vi "测试-Z值判定.vi"() -> ()   [LabVIEW 2018]
uses:
  <vilib>/Utility/NIReport.llb/Report Type.ctl
  <vilib>/Utility/NIReport.llb/Append Report Text (str wrap).vi
  <vilib>/addons/_office/word.llb/Word Edit Cell (str).vi
  <vilib>/Utility/NIReport.llb/NI_report.lvclass
  <vilib>/Utility/NIReport.llb/NI_ReportGenerationCore.lvlib
  <vilib>/Utility/NIReport.llb/Word/NI_Word.lvclass
  <vilib>/addons/_office/NI_ReportGenerationToolkit.lvlib
panel:
  out "报告生成路径":path
  in  "产品序号":string
  out "字符串":string
  in  "Z值":dbl[](array[numeric])
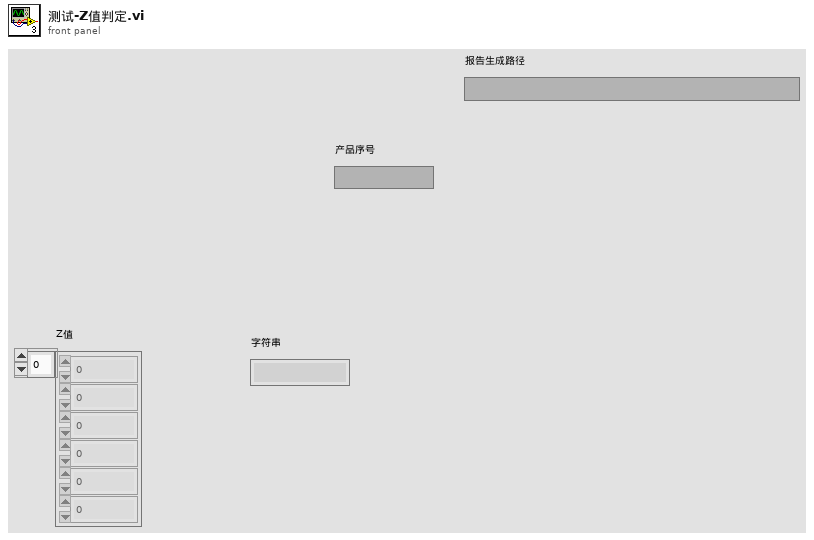
[diagram p1: front panel]
types:
  T1 = cluster{"position (Excel)":cluster{"row":i32, "column":i32}, "name (Excel)":string, "bookmark (Word)":string}
  T2 = typedef "NI_ReportGenerationCore.lvlib/Report Type.ctl" = enum16{"HTML", "Word", "Excel"}
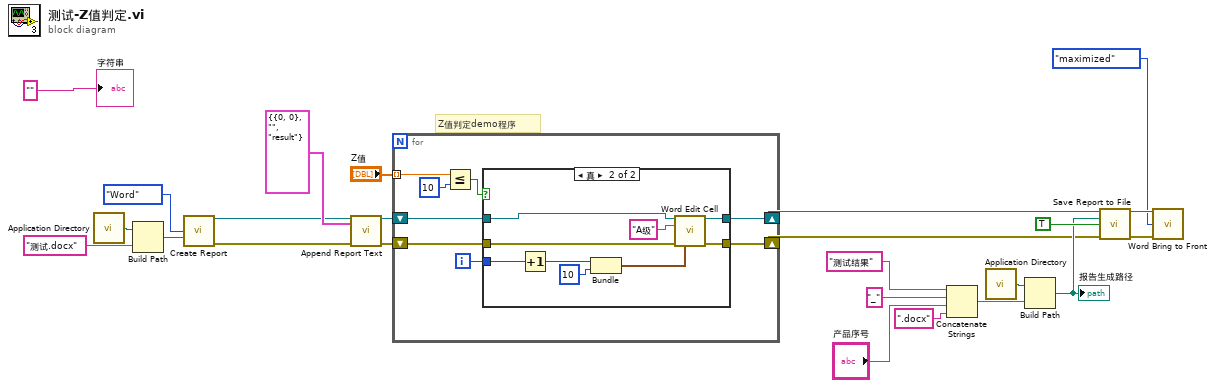
[diagram p0: block diagram]
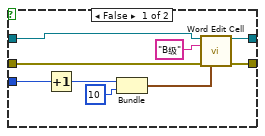
[diagram p2: hidden frame]
diagram:
  # "Z值判定demo程序"
  n1 = call <vilib>:"Application Directory.vi"() -> ("Application Directory"=w21:path)
  n2 = Build Path(base path=w21, name or relative path="测试.docx") -> (appended path=w24:path)
  n3 = call <vilib>:"Create Report.vi"("report type"=Report_Type."Word" ("Report Type"), "template (empty)"=w24) -> ("report out"=w6:refnum<class "NI_report.lvclass">, "error out"=w5:errorcluster)  [unwired: 12 in]
  n4 = call-poly <vilib>:"Append Report Text.vi"("report in"=w6, "MS Office parameters"=T1 {"position (Excel)"={"row"=0, "column"=0}, "name (Excel)"="", "bookmark (Word)"="result"}, "error in (no error)"=w5) -> ("report out"=w3:refnum<class "NI_report.lvclass">, "error out"=w4:errorcluster)  [unwired: 9 in, 2 out]
  n5 = for {
    shift-right: [w25] -> w2
    shift-left: w3 -> [w28]
    shift-right: [w26] -> w1
    shift-left: w4 -> [w27]
    tunnel: "Z值" -> [w31] mode=indexing
    i -> [w29]
    n6 = Less Or Equal?(x=w31, y=10) -> (x <= y?=w30:bool)
    n7 = case shown="真" w30 {
      tunnel: w29 -> [w35 w48]
      tunnel: w28 -> [w36 w47]
      tunnel: w27 -> [w37 w46]
      tunnel: [w34 w45] -> w26
      tunnel: [w33 w44] -> w25
      frame False {
        n8 = Increment(x=w35) -> (x+1=w41:i32)
        n9 = Bundle(w41, "y"=10) -> (w38:cluster{i32, "y":i32})  [unwired: 1 in]
        n10 = call-poly <vilib>:"Word Edit Cell.vi"("report in"=w36, "value"="B级", "error in (no error)"=w37, "start (0, 0)"=w38) -> ("report out"=w33:refnum<class "NI_report.lvclass">, "error out"=w34:errorcluster)  [unwired: 10 in]
      }
      frame True {
        n11 = Increment(x=w48) -> (x+1=w50:i32)
        n12 = Bundle(w50, "y"=10) -> (w42:cluster{i32, "y":i32})  [unwired: 1 in]
        n13 = call-poly <vilib>:"Word Edit Cell.vi"("report in"=w47, "value"="A级", "error in (no error)"=w46, "start (0, 0)"=w42) -> ("report out"=w44:refnum<class "NI_report.lvclass">, "error out"=w45:errorcluster)  [unwired: 10 in]
      }
    }
  }
  n14 = Concatenate Strings("测试结果" ("字符串"), "_" ("名称或相对路径"), "产品序号", ".docx" ("名称或相对路径")) -> (w11:string)
  n15 = call <vilib>:"Application Directory.vi"() -> ("Application Directory"=w10:path)
  n16 = Build Path(base path=w10, name or relative path=w11) -> (appended path=w8:path)
  "报告生成路径" <- w8
  n17 = call-dynamic "Save Report to File.vi"("report in"=w2, "report file path"=w8, "prompt to replace? (F)"=TRUE, "error in (no error)"=w1) -> ("report out"=w16:refnum<class "NI_report.lvclass">, "error out"=w17:errorcluster)  [unwired: 10 in]
  n18 = call <vilib>:"Word Bring to Front.vi"("report in"=w16, "window state (maximized)"=enum16{"maximized", "minimized", "normal"}."maximized", "error in (no error)"=w17) -> ()  [unwired: 11 in, 2 out]
  "字符串" <- ""
